vi "Comm String Flush Port.vi"(0 "niDTS Comm Serial in":refnum<class "niDTS Comm Serial.lvclass">, 7 "Read Data (F)":bool, 9 "Log Data (F)":bool, 11 "error in (no error)":errorcluster) -> (4 "niDTS Comm Serial out":refnum<class "niDTS Comm Serial.lvclass">, 8 "Read Data":string, 15 "error out":errorcluster)   [LabVIEW 2015, in "niDTS CommLib.lvlib" / "niDTS Comm Serial.lvclass"]
uses:
  niDTS Comm Serial.lvclass
  Dependencies/__VISA Flush IO Buffer Mask.ctl
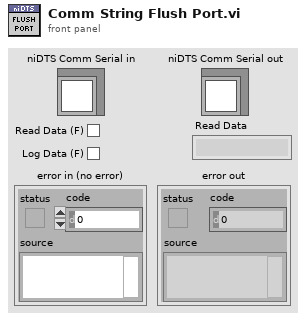
[diagram p1: front panel]
types:
  T1 = typedef "__VISA Flush IO Buffer Mask.ctl" = u16
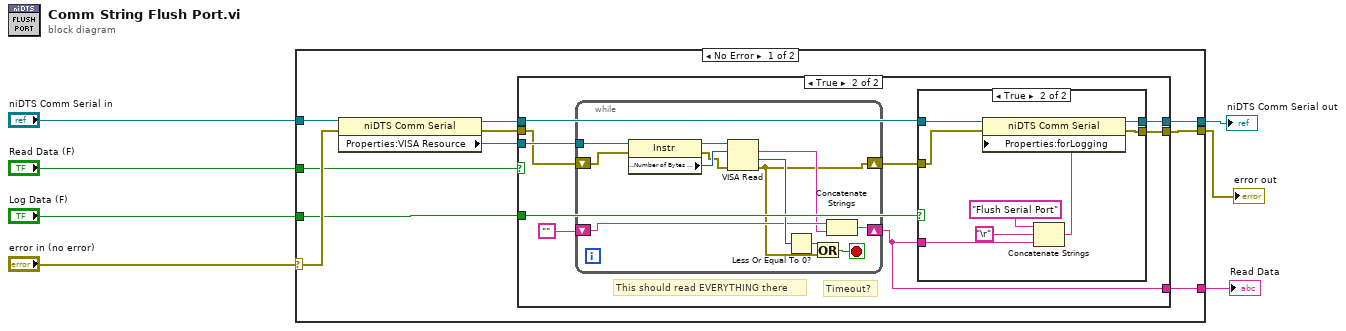
[diagram p0: block diagram]
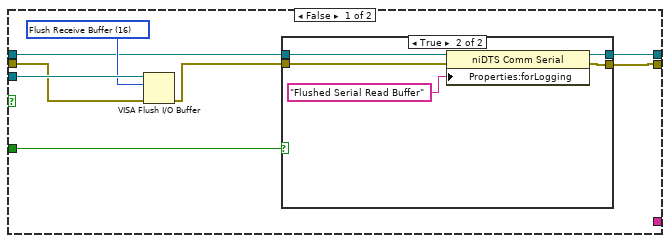
[diagram p2: hidden frame]
diagram:
  n1 = case shown="No Error" "error in (no error)" {
    selector: "error in (no error)" -> [w16 w64]
    tunnel: "Log Data (F)" -> [w11 _]
    tunnel: "Read Data (F)" -> [w15 _]
    tunnel: "niDTS Comm Serial in" -> [w17 w65]
    tunnel: [w10 w65] -> w3
    tunnel: [w9 _] -> w2
    tunnel: [w8 w64] -> w1
    frame No Error {
      n2 = property class="niDTS Comm Serial"(reference=w17, error in=w16) -> (reference out=w12:refnum<class "niDTS Comm Serial.lvclass">, error out=w13:errorcluster, "Properties:VISA Resource"=w14:refnum<visa-resource-name>)
      n3 = case shown="True" w15 {
        tunnel: w14 -> [w25 w41]
        tunnel: w13 -> [w24 w39]
        tunnel: w12 -> [w22 w37]
        tunnel: w11 -> [w21 w38]
        tunnel: [w19 w35] -> w10
        tunnel: [_ w34] -> w9
        tunnel: [w18 w33] -> w8
        frame False {
          w23 = T1 16 items=["Flush Receive Buffer"=16, "Write Transmit Buffer to Device"=32, "Flush Receive Buffer (No I/O)"=64, "Flush Transmit Buffer"=128] ("Mask")
          n4 = VISA Flush I/O Buffer(VISA resource name=w25, mask (16)=w23, error in (no error)=w24) -> (error out=w20:errorcluster)  [unwired: 1 out]
          n5 = case shown="True" w21 {
            tunnel: w22 -> [w27 w32]
            tunnel: w20 -> [w26 w30]
            tunnel: [w27 w29] -> w19
            tunnel: [w26 w28] -> w18
            frame False {
            }
            frame True {
              n6 = property class="niDTS Comm Serial"(reference=w32, error in=w30, "Properties:forLogging"="Flushed Serial Read Buffer" ("forLogging")) -> (reference out=w29:refnum<class "niDTS Comm Serial.lvclass">, error out=w28:errorcluster)
            }
          }
        }
        frame True {
          # "Timeout?"
          # "This should read EVERYTHING there"
          n7 = while {
            tunnel: w41 -> [w61]
            shift-right: [w57] -> w34
            shift-left: "" -> [w56]
            shift-right: [w52] -> w36
            shift-left: w39 -> [w53]
            stop <- w58 stop-if-true
            n8 = property class="Instr"(reference=w61, error in=w53) -> (reference out=w54:refnum<visa-resource-name>, error out=w62:errorcluster, "Serial Settings:Number of Bytes at Serial Port"=w63:u32)
            n9 = VISA Read(VISA resource name=w54, byte count=w63, error in (no error)=w62) -> (read buffer=w55:string, return count=w60:u32, error out=w52:errorcluster)  [unwired: 1 out]
            n10 = Less Or Equal To 0?(x=w60) -> (x <= 0?=w59:bool)
            n11 = Or(x=w59, y=w52) -> (x .or. y?=w58:bool)
            n12 = Concatenate Strings(w56, w55) -> (w57:string)
          }
          n13 = case shown="True" w38 {
            tunnel: w37 -> [w43 w48]
            tunnel: w36 -> [w42 w47]
            tunnel: w34 -> [_ w46]
            tunnel: [w43 w45] -> w35
            tunnel: [w42 w44] -> w33
            frame False {
            }
            frame True {
              n14 = Concatenate Strings("Flush Serial Port", "\r", w46) -> (w51:string)
              n15 = property class="niDTS Comm Serial"(reference=w48, error in=w47, "Properties:forLogging"=w51) -> (reference out=w45:refnum<class "niDTS Comm Serial.lvclass">, error out=w44:errorcluster)
            }
          }
        }
      }
    }
    frame Error {
    }
  }
  "error out" <- w1
  "niDTS Comm Serial out" <- w3
  "Read Data" <- w2
